vi "탭웹브라우저_noloop.vi"() -> ()   [LabVIEW 2014]
panel:
  in  "WebBrowser":refnum<k7>(container)
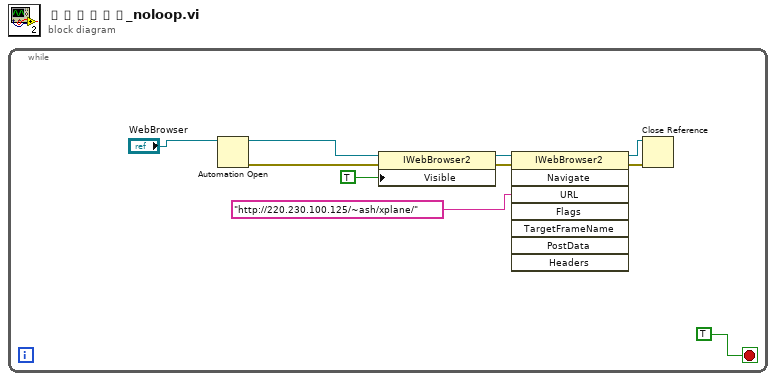
[diagram p0: block diagram]
diagram:
  n1 = while {
    stop <- TRUE stop-if-true
    n2 = Automation Open(Automation Refnum="WebBrowser") -> (Automation Refnum=w7:refnum<k7>, error out=w6:errorcluster)  [unwired: 1 in, 2 out]
    n3 = property class="IWebBrowser2"(reference=w7, error in=w6, "Visible"=TRUE) -> (reference out=w8:refnum<k7>, error out=w9:errorcluster)
    n4 = invoke class="IWebBrowser2" method="Navigate"(reference=w8, error in=w9, "URL"="http://220.230.100.125/~ash/xplane/") -> (reference out=w4:refnum<k7>, error out=w5:errorcluster)  [unwired: 5 in, 6 out]
    n5 = Close Reference(reference=w4, error in (no error)=w5) -> ()  [unwired: 1 out]
  }
